vi "(,,,) FROM.vi"(10 "Column Names":string[](array[string])=["Col1", "Col2", "Col3"], 11 "SQL containing FROM clause":string="SELECT FROM TableA") -> (3 "SQL":string caption="SQL with colums inserted before FROM")   [LabVIEW 2011, in "SQLite.lvlib"]
doc: "Formats an array of column names before the \"FROM\" keyword in the input SQL INSERT statement. For use when working with a dynamically list of columns."
uses:
  SQLite.lvlib
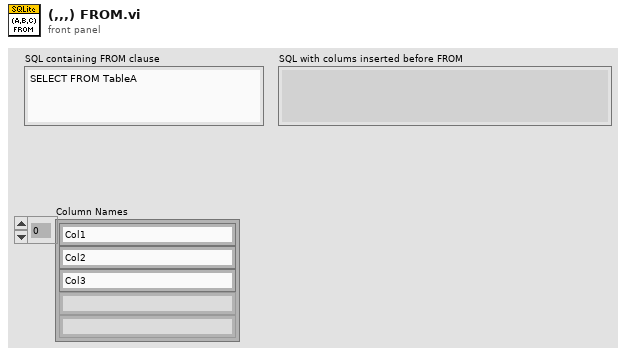
[diagram p1: front panel]
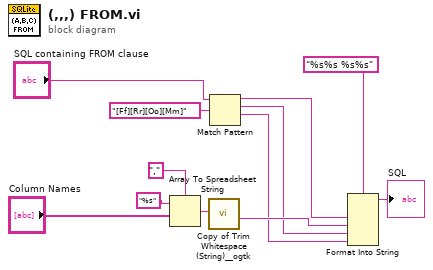
[diagram p0: block diagram]
diagram:
  n1 = Array To Spreadsheet String(delimiter (Tab)=",", array="Column Names", 3:"%s" ("format string")) -> (spreadsheet string=w10:string)
  n2 = call "Copy of Trim Whitespace (String)__ogtk.vi"("String in"=w10) -> ("String out"=w3:string)  [unwired: 6 in]
  n3 = Match Pattern(string="SQL containing FROM clause", regular expression="[Ff][Rr][Oo][Mm]") -> (before substring=w4:string, match substring=w2:string, after substring=w1:string)  [unwired: 1 in, 1 out]
  n4 = Format Into String(format string="%s%s %s%s", w4, w3, w2, w1) -> (resulting string=→"SQL":string)  [unwired: 2 in, 1 out]
